vi "Test MultiValue INSERT format.vi"() -> ()   [LabVIEW 2019, in "LV-Data.PGSQL.lvclass"]
uses:
  LV-Data.PGSQL.lvclass
panel:
  out "Data":string[](array[string])
  in  "String":string
  in  "Data (array)":string[](array[string])=["", ""]
  in  "Data (array of cluster)":cluster{"Numeric 2":dbl}[](array[cluster])=[{"Numeric 2"=-1.0}, {"Numeric 2"=-2.0}]
  in  "Timestamps":timestamp[](array[timestamp])=[timestamp(3753094947.978874 s since 1904-01-01), timestamp(3753094950.8230257 s since 1904-01-01), timestamp(3810819142.718672 s since 1904-01-01)]
  in  "Data (multi multirow)":T1(array[cluster])=[{"String"="string 1", "Numeric"=1.0, "Numeric 2"=2.0}, {"String"="string 2", "Numeric"=3.0, "Numeric 2"=4.0}, {"String"="string 3", "Numeric"=5.0, "Numeric 2"=6.0}]
  in  "path(s)":string[](array[string])=["llab_025:v001(Montana Cryostation--User())", "llab_025:d008(Montana Cryostation--Cold Head Speed(Hz))", "llab_061:d000(AML Gauges (Analysis)--IG Pressure(mbar))"]
  out "Formatted Insert":string="INSERT INTO\n  llab_025 (d008,time,v001)\nVALUES\n  (1,'2022-12-05 09:22:27.978874'::timestamptz,$$string 1$$),\n  (3,'2022-12-05 09:22:30.823025'::timestamptz,$$string 2$$),\n  (5,'2024-10-03 12:52:22.718671'::timestamptz,$$string 3$$)\r\n;\nINSERT INTO\n  llab_061 (d000,time)\nVALUES\n  (2,'2022-12-05T14:22:27.978Z'::timestamptz),\n  (4,'2022-12-05T14:22:30.823Z'::timestamptz),\n  (6,'2024-10-03T16:52:22.718Z'::timestamptz)\r\n;"
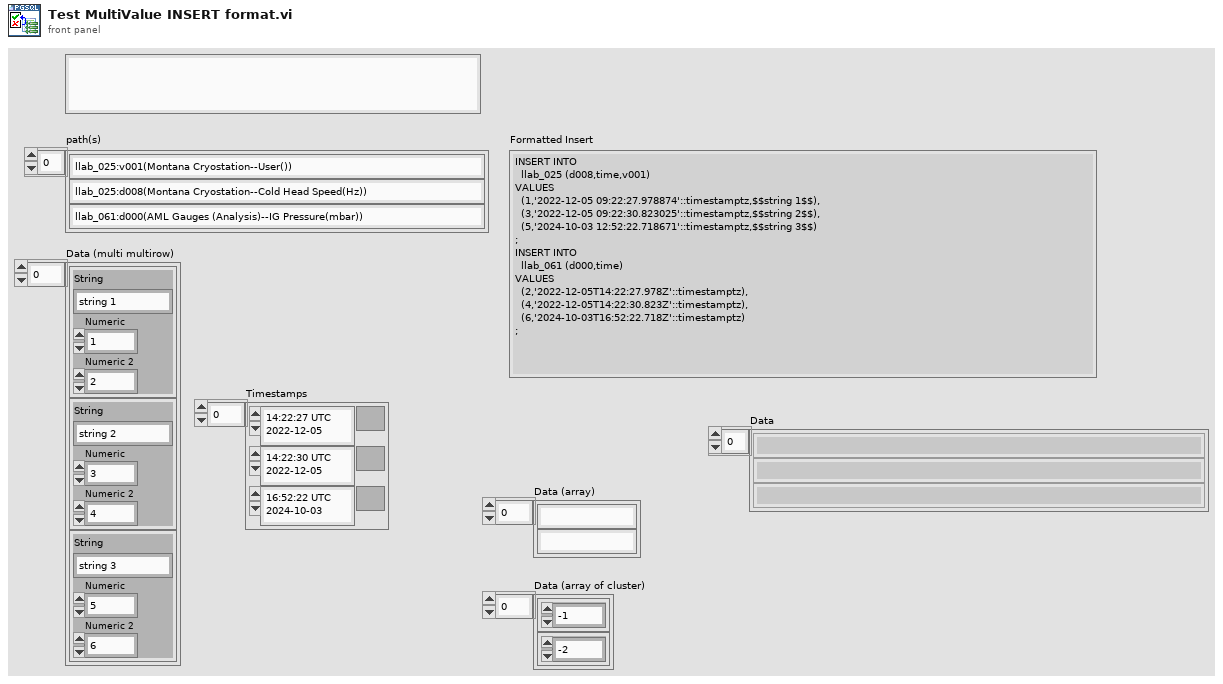
[diagram p1: front panel]
types:
  T1 = cluster{"String":string, "Numeric":dbl, "Numeric 2":dbl}[]
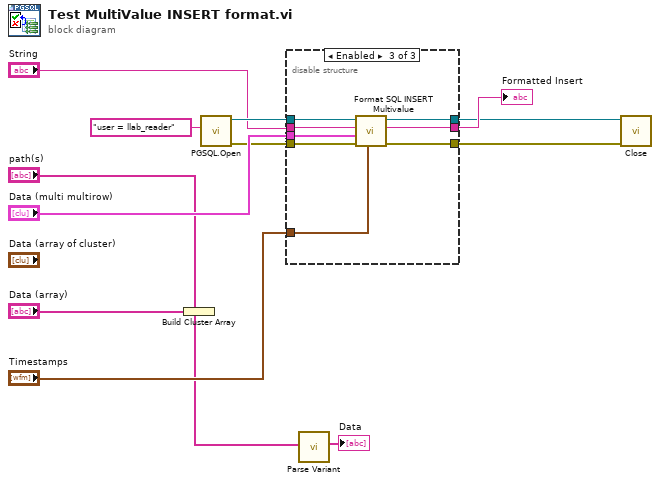
[diagram p0: block diagram]
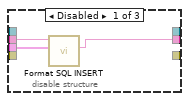
[diagram p2: hidden frame]
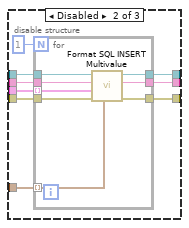
[diagram p3: hidden frame]
diagram:
  n1 = Build Cluster Array("Data (array)") -> ()  [unwired: 1 out]
  n2 = call "PGSQL.Open.vi"("Connection String"="user = llab_reader") -> ("error out"=w5:errorcluster, "Data.PG out"=w9:refnum<class "LV-Data.PGSQL.lvclass">)  [unwired: 9 in]
  n3 = disable-structure shown="Enabled" {
    disable-tunnel: [w15 w24 w35] -> w12
    disable-tunnel: "String" -> [w14 w23 w38]
    disable-tunnel: "Data (multi multirow)" -> [w13 w22 w37]
    disable-tunnel: "Timestamps" -> [_ w21 w36]
    disable-tunnel: w9 -> [_ w20 w40]
    disable-tunnel: [_ w19 w39] -> w7
    disable-tunnel: w5 -> [_ w18 w33]
    disable-tunnel: [_ w17 w34] -> w4
    frame Disabled {
      n4 = call "Format SQL INSERT.vi"("Data"=w13, "Path(s)"=w14) -> ("Formatted Insert"=w15:string)  [unwired: 7 in, 2 out]
    }
    frame Disabled {
      n5 = for {
        N: 1 -> [_]
        tunnel: [w32] -> w24
        tunnel: w23 -> [w31]
        tunnel: w22 -> [w30] mode=indexing
        tunnel: w21 -> [w29] mode=indexing
        tunnel: w20 -> [w28]
        tunnel: [w27] -> w19
        tunnel: w18 -> [w26]
        tunnel: [w25] -> w17
        n6 = call "Format SQL INSERT Multivalue.vi"("Times"=w29, "error in"=w26, "Data"=w30, "Path(s)"=w31, "Data.PG in"=w28) -> ("error out"=w25:errorcluster, "SQL"=w32:string, "Data.PG out"=w27:refnum<class "LV-Data.PGSQL.lvclass">)  [unwired: 3 in, 1 out]
      }
    }
    frame Enabled {
      n7 = call "Format SQL INSERT Multivalue.vi"("Times"=w36, "error in"=w33, "Data"=w37, "Path(s)"=w38, "Data.PG in"=w40) -> ("error out"=w34:errorcluster, "SQL"=w35:string, "Data.PG out"=w39:refnum<class "LV-Data.PGSQL.lvclass">)  [unwired: 3 in, 1 out]
    }
  }
  "Formatted Insert" <- w12
  n8 = call "Parse Variant.vi"("Data"="path(s)") -> ("Data"=→"Data":string[])  [unwired: 6 in, 4 out]
  n9 = call-dynamic "Close.vi"("error in (no error)"=w4, "Data.PG in"=w7) -> ()  [unwired: 8 in, 2 out]
